vi "Matriz 2x2.vi"() -> ()   [LabVIEW 2020]
uses:
  <vilib>/numeric/Random Number (Range) U64.vi
  <vilib>/numeric/sub_Random U32.vi
panel:
  in  "Indicador fila":i32=3
  in  "Indicador columna":i32=3
  out "Resultado":dbl
  out "size(s)":i32[](array[numeric])
  in  "Columnas":i32
  in  "Filas":i32=5
  out "Tabla de multiplicar":dbl[][](array[numeric])
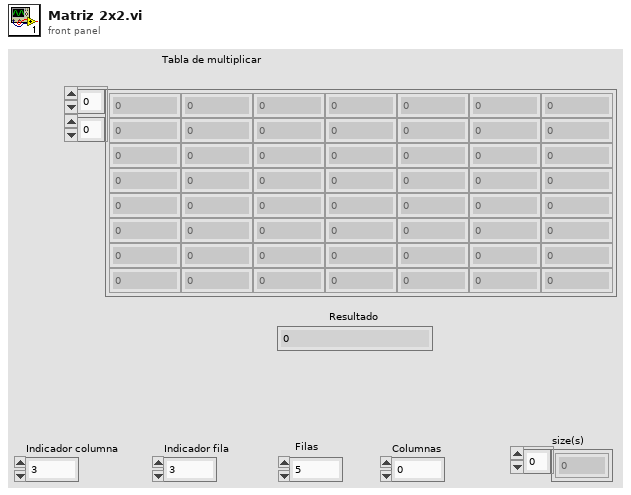
[diagram p1: front panel]
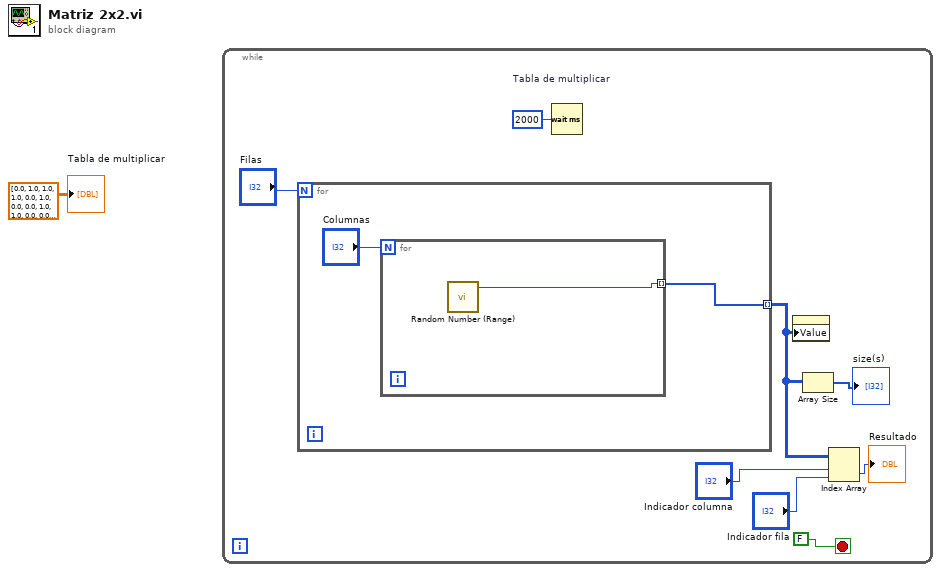
[diagram p0: block diagram]
diagram:
  n1 = while {
    stop <- FALSE stop-if-true
    n2 = for {
      N: "Filas" -> [_]
      tunnel: [w11] -> w5 mode=indexing
      n3 = for {
        N: "Columnas" -> [_]
        tunnel: [w12] -> w11 mode=indexing
        n4 = call-poly <vilib>:"Random Number (Range).vi"() -> ("number"=w12:u64)  [unwired: 11 in]
      }
    }
    n5 = Wait (ms)(milliseconds to wait=u32 2000) -> ()  [unwired: 1 out]
    n6 = property on="Tabla de multiplicar" class="Arr (strict)"("Value"=w5) -> ()  [unwired: 2 in, 2 out]
    n7 = Array Size(array=w5) -> (size(s)=→"size(s)":i32[])
    n8 = Index Array(array=w5, index (row)="Indicador columna", index (col)="Indicador fila") -> (element=→"Resultado":u64)
  }
  "Tabla de multiplicar" <- dbl[][] [[0.0, 1.0, 1.0, 1.0, 0.0], [1.0, 0.0, 0.0, 1.0, 1.0], [0.0, 0.0, 1.0, 1.0, 0.0], [0.0, 0.0, 1.0, 0.0, 1.0], [1.0, 0.0, 0.0, 1.0, 0.0], [1.0, 0.0, 1.0, 1.0, 0.0], [1.0, 0.0, 1.0, 0.0, 0.0]] ("Array")
